vi "AutoTurnToHot.vi"(8 "error in (no error)":errorcluster, 10 "Left/Right":enum16{"Left", "Right", ""}(ring), 11 "Hot?":bool) -> (0 "error out":errorcluster)   [LabVIEW 2013]
uses:
  AutoTurnToHotStates.ctl
  ShooterStates.ctl
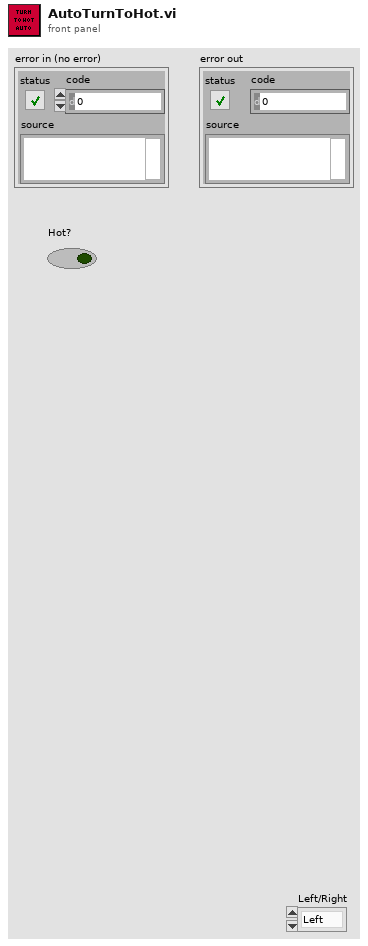
[diagram p1: front panel]
types:
  T1 = typedef "AutoTurnToHotStates.ctl" = enum16{"Check Hot", "Turn", "Fire", "Drive Forward"}
  T2 = typedef "ShooterStates.ctl" = enum16{"Ready", "Fire", "Fire Delay", "Latch", "Retract"}
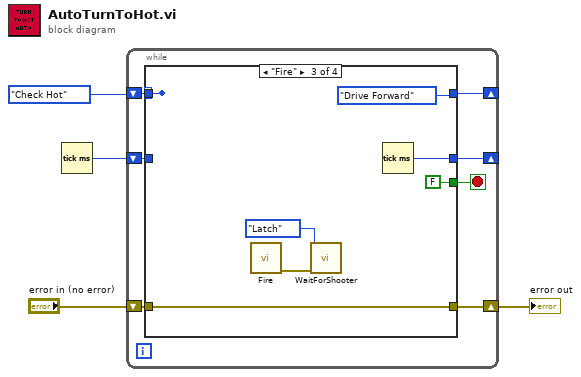
[diagram p0: block diagram]
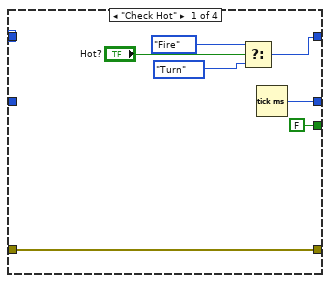
[diagram p2: hidden frame]
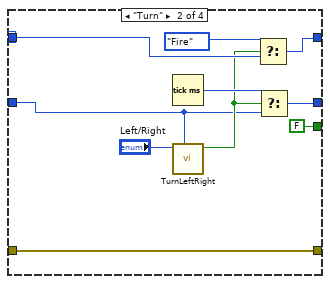
[diagram p3: hidden frame]
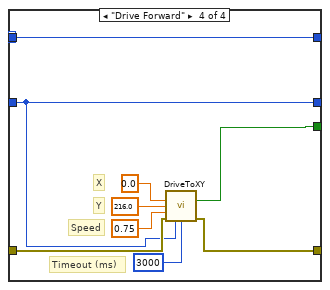
[diagram p4: hidden frame]
diagram:
  n1 = Tick Count (ms)() -> (millisecond timer value=w4:u32)
  n2 = while {
    shift-right: [w10] -> w3
    shift-left: "error in (no error)" -> [w11]
    shift-right: [w8] -> _
    shift-left: w4 -> [w9]
    shift-right: [w5] -> _
    shift-left: AutoTurnToHotStates."Check Hot" -> [w6]
    stop <- w7 stop-if-true
    n3 = case shown="\"Fire\"" w6 {
      selector: w6 -> [_ w26 _ w35]
      tunnel: w11 -> [w14 w24 w34 w40]
      tunnel: [w14 w24 w34 w39] -> w10
      tunnel: [w17 w25 AutoTurnToHotStates."Drive Forward" w35] -> w5
      tunnel: w9 -> [_ w19 _ w37]
      tunnel: [w16 w27 w29 w37] -> w8
      tunnel: [FALSE FALSE FALSE w36] -> w7
      tunnel: w6 -> [_ _ _ _]
      frame "Check Hot" {
        n4 = Select(t=AutoTurnToHotStates."Fire", s="Hot?", f=AutoTurnToHotStates."Turn") -> (s? t:f=w17:T1)
        n5 = Tick Count (ms)() -> (millisecond timer value=w16:u32)
      }
      frame "Turn" {
        n6 = Tick Count (ms)() -> (millisecond timer value=w28:u32)
        n7 = call "TurnLeftRight.vi"("Start time"=w19, "Left/Right"="Left/Right") -> ("Done"=w20:bool)  [unwired: 9 in]
        n8 = Select(t=AutoTurnToHotStates."Fire", s=w20, f=w26) -> (s? t:f=w25:T1)
        n9 = Select(t=w28, s=w20, f=w19) -> (s? t:f=w27:u32)
      }
      frame "Fire" {
        n10 = call "Fire.vi"() -> ("error out"=w32:errorcluster)  [unwired: 11 in]
        n11 = call "WaitForShooter.vi"("error in (no error)"=w32, "State"=ShooterStates."Latch") -> ()  [unwired: 8 in, 2 out]
        n12 = Tick Count (ms)() -> (millisecond timer value=w29:u32)
      }
      frame "Drive Forward" {
        # "Timeout (ms)"
        # "Speed"
        # "Y"
        # "X"
        n13 = call "DriveToXY.vi"("X Target"=0.0, "Y Target"=216.0, "Speed"=0.75, "error in"=w40, "Start time"=w37, "Timeout (ms)"=u32 3000 ("y")) -> ("At Target"=w36:bool, "error out"=w39:errorcluster)  [unwired: 6 in, 2 out]
      }
    }
  }
  "error out" <- w3
